vi "ASW(SubVI).vi"(8 "error in (no error)":errorcluster) -> (0 "error out":errorcluster, 1 "ASW(TS)":dbl[](array[numeric]), 2 "ASW(KN)":dbl[](array[numeric]), 3 "ASW(ZN)":dbl[](array[numeric]))   [LabVIEW 2019]
uses:
  Global.vi
  <vilib>/express/express arith-compare/Formula/XNode/ExpressFormulaBlockNode.xnode
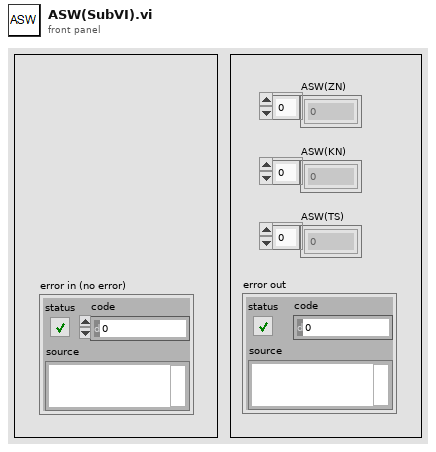
[diagram p1: front panel]
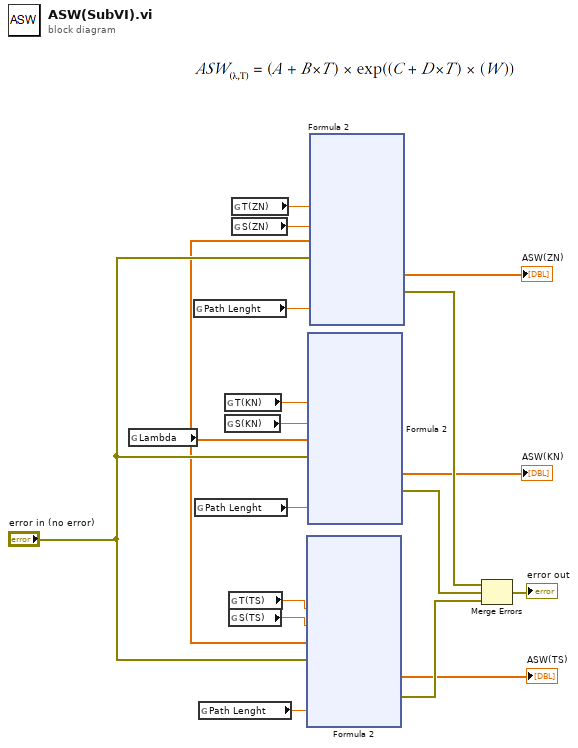
[diagram p0: block diagram]
diagram:
  n1 = global read "Global.vi" "Lambda"() -> (w4:dbl[])
  n2 = global read "Global.vi" "Path Lenght"() -> (w3:dbl)
  n3 = global read "Global.vi" "Path Lenght"() -> (w1:dbl)
  n4 = global read "Global.vi" "Path Lenght"() -> (w2:dbl)
  n5 = global read "Global.vi" "T(KN)"() -> (w8:dbl)
  n6 = global read "Global.vi" "S(KN)"() -> (w7:dbl)
  n7 = global read "Global.vi" "T(TS)"() -> (w6:dbl)
  n8 = global read "Global.vi" "S(TS)"() -> (w5:dbl)
  n9 = global read "Global.vi" "T(ZN)"() -> (w10:dbl)
  n10 = global read "Global.vi" "S(ZN)"() -> (w9:dbl)
  n11 = xnode "Formula 2"("T"=w6, "S"=w5, "W"=w4, "error in (no error)"="error in (no error)", "P"=w2) -> ("Result"=→"ASW(TS)":dbl[], "error out"=w17:errorcluster)
  n12 = xnode "Formula 2"("T"=w8, "S"=w7, "W"=w4, "error in (no error)"="error in (no error)", "P"=w1) -> ("Result"=→"ASW(KN)":dbl[], "error out"=w13:errorcluster)
  n13 = xnode "Formula 2"("T"=w10, "S"=w9, "W"=w4, "error in (no error)"="error in (no error)", "P"=w3) -> ("Result"=→"ASW(ZN)":dbl[], "error out"=w14:errorcluster)
  n14 = Merge Errors(w14, w13, w17) -> (→"error out":errorcluster)
